vi "different_length.vi"(8 "newY":dbl, 9 "newX":dbl, 10 "pY":dbl, 11 "pX":dbl) -> (0 "dY":dbl, 1 "dX":dbl, 2 "dirY":bool[](array[boolean]), 3 "dirX":bool[](array[boolean]))   [LabVIEW 2016]
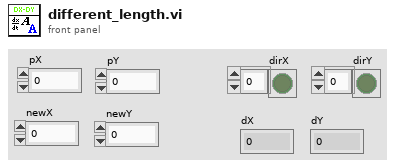
[diagram p1: front panel]
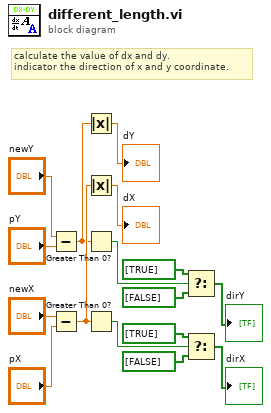
[diagram p0: block diagram]
diagram:
  # "calculate the value of dx and dy.\nindicator the direction of x and y coordinate."
  n1 = Subtract(x="newY", y="pY") -> (x-y=w11:dbl)
  n2 = Subtract(x="newX", y="pX") -> (x-y=w12:dbl)
  n3 = Absolute Value(x=w11) -> (abs(x)=→"dY":dbl)
  n4 = Absolute Value(x=w12) -> (abs(x)=→"dX":dbl)
  n5 = Greater Than 0?(x=w11) -> (x > 0?=w7:bool)
  n6 = Greater Than 0?(x=w12) -> (x > 0?=w13:bool)
  n7 = Select(t=bool[] [TRUE], s=w7, f=bool[] [FALSE]) -> (s? t:f=→"dirY":bool[])
  n8 = Select(t=bool[] [TRUE], s=w13, f=bool[] [FALSE]) -> (s? t:f=→"dirX":bool[])
